vi "PH_SSAC.ProcEvents.vi"(0 "i ref in":refnum<vi>, 5 "error in":errorcluster) -> (14 "i ref out":refnum<vi>, 19 "error out":errorcluster)   [LabVIEW 2014, in "PH_SSAC.lvlib"]
doc: "This method is used to define the events the object will listen to. Add your own events here."
uses:
  PH_SSAC.lvlib
  CSCore/BaseProcess/BaseProcess.event definition.ctl
  CSCore/CAEObj/CAEObj.event definition.ctl
  CSCore/BaseProcess/BaseProcess.descriptor string definition.ctl
  CSCore/BaseProcess/BaseProcess.lvlib
  CSCore/CAEObj/CAEObj.lvlib
  PH_Common/PH_Common.lvlib
  PH_Img_BaseClass/PH_Img_BaseClass.lvlib
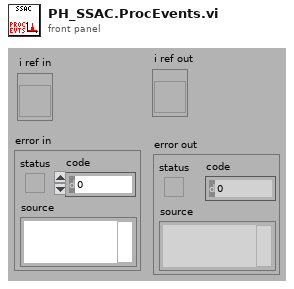
[diagram p1: front panel]
types:
  T1 = typedef "BaseProcess.lvlib/BaseProcess.event definition.ctl" = cluster{"CAEEvtDef":T2, "Data Descriptor":T3}
  T2 = typedef "CAEObj.lvlib/CAEObj.event definition.ctl" = cluster{"URL":string, "enable":bool, "ignoreResID":bool}
  T3 = typedef "BaseProcess.lvlib/BaseProcess.descriptor string definition.ctl" = string
  T4 = typedef "PH_Img_BaseClass.lvlib/PH_Img_BaseClass.i attribute.ctl" = cluster{"GUI Refs":T5, "Timeout Image [ms]":i32, "Default Periodic Period [ms]":i32, "Camera":cluster{"Instancename":string, "Notifier":refnum<notifier>}, "Palette":T6, "Cam Settings":cluster{"Cam ID":string, "Gain":dbl, "Brightness":dbl, "Shutter":dbl, "Cam Info Failure":bool, "Mode":i32}}
  T5 = typedef "PH_Img_BaseClass.lvlib/PH_Img_BaseClass.GUI Refs.ctl" = cluster{"Timeout":refnum<vi>, "Image":refnum<vi>, "Palette":refnum<vi>, "Timeout Set":refnum<vi>}
  T6 = typedef "PH_Img_BaseClass.lvlib/PH_Img_BaseClass.Palette.ctl" = i32
  T7 = typedef "PH_Common.lvlib/PH_DIM.Event Declarer.ctl" = cluster{"Service Name":string, "Selector":string}
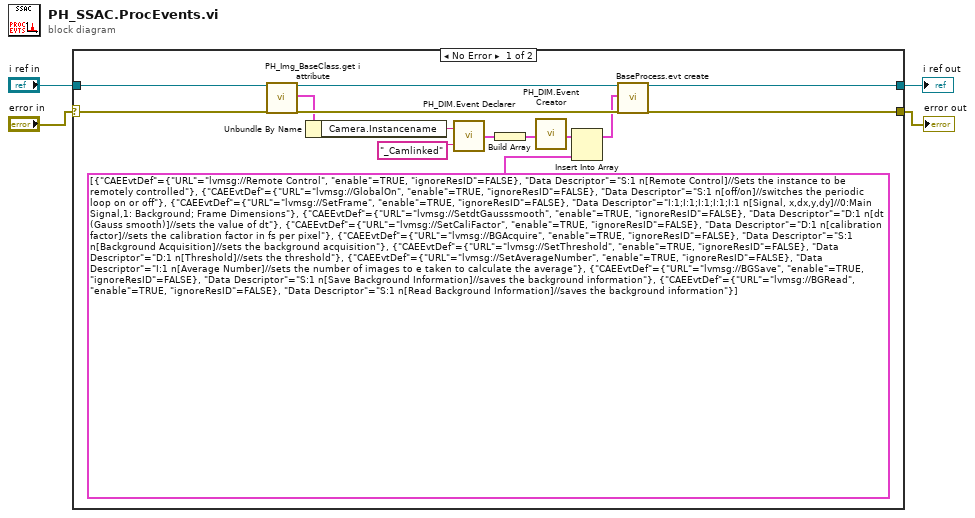
[diagram p0: block diagram]
diagram:
  n1 = case shown="No Error" "error in" {
    selector: "error in" -> [w16 w19]
    tunnel: "i ref in" -> [w14 w20]
    tunnel: [w18 w20] -> w3
    tunnel: [w17 w19] -> w2
    frame No Error {
      n2 = call "PH_Img_BaseClass.get i attribute.vi"("i ref in"=w14, "error in (no error)"=w16) -> ("i ref out"=w13:refnum<vi>, "i attribute"=w12:T4, "error out"=w15:errorcluster)  [unwired: 15 in]
      n3 = Unbundle By Name(w12) -> ("Camera.Instancename"=w7:string)
      n4 = call "PH_DIM.Event Declarer.vi"("Selector"="_Camlinked" ("URL"), "Service Name"=w7) -> ("declared DIM Event"=w8:T7)
      n5 = Build Array(w8) -> (w5:T7[])
      n6 = call "PH_DIM.Event Creator.vi"("condition Services"=w5) -> ("DIM Service Events"=w9:T1[])  [unwired: 18 in]
      n7 = Insert Into Array(array=w9, new element=T1[] [{"CAEEvtDef"={"URL"="lvmsg://Remote Control", "enable"=TRUE, "ignoreResID"=FALSE}, "Data Descriptor"="S:1 n[Remote Control]//Sets the instance to be remotely controlled"}, {"CAEEvtDef"={"URL"="lvmsg://GlobalOn", "enable"=TRUE, "ignoreResID"=FALSE}, "Data Descriptor"="S:1 n[off/on]//switches the periodic loop on or off"}, {"CAEEvtDef"={"URL"="lvmsg://SetFrame", "enable"=TRUE, "ignoreResID"=FALSE}, "Data Descriptor"="I:1;I:1;I:1;I:1;I:1 n[Signal, x,dx,y,dy]//0:Main Signal,1: Background; Frame Dimensions"}, {"CAEEvtDef"={"URL"="lvmsg://SetdtGausssmooth", "enable"=TRUE, "ignoreResID"=FALSE}, "Data Descriptor"="D:1 n[dt (Gauss smooth)]//sets the value of dt"}, {"CAEEvtDef"={"URL"="lvmsg://SetCaliFactor", "enable"=TRUE, "ignoreResID"=FALSE}, "Data Descriptor"="D:1 n[calibration factor]//sets the calibration factor in fs per pixel"}, {"CAEEvtDef"={"URL"="lvmsg://BGAcquire", "enable"=TRUE, "ignoreResID"=FALSE}, "Data Descriptor"="S:1 n[Background Acquisition]//sets the background acquisition"}, {"CAEEvtDef"={"URL"="lvmsg://SetThreshold", "enable"=TRUE, "ignoreResID"=FALSE}, "Data Descriptor"="D:1 n[Threshold]//sets the threshold"}, {"CAEEvtDef"={"URL"="lvmsg://SetAverageNumber", "enable"=TRUE, "ignoreResID"=FALSE}, "Data Descriptor"="I:1 n[Average Number]//sets the number of images to e taken to calculate the average"}, {"CAEEvtDef"={"URL"="lvmsg://BGSave", "enable"=TRUE, "ignoreResID"=FALSE}, "Data Descriptor"="S:1 n[Save Background Information]//saves the background information"}, {"CAEEvtDef"={"URL"="lvmsg://BGRead", "enable"=TRUE, "ignoreResID"=FALSE}, "Data Descriptor"="S:1 n[Read Background Information]//saves the background information"}] ("new events")) -> (w11:T1[])  [unwired: 1 in]
      n8 = call "BaseProcess.evt create.vi"("i ref in"=w13, "newEvents"=w11, "error in (no error)"=w15) -> ("i ref out"=w18:refnum<vi>, "error out"=w17:errorcluster)  [unwired: 13 in, 2 out]
    }
    frame Error {
    }
  }
  "i ref out" <- w3
  "error out" <- w2
